vi "gbtpFit.vi"(6 "Y":dbl[](array[numeric]), 8 "error in (no error)":errorcluster, 9 "termination":cluster{"max iteration":i32, "tolerance":dbl}, 10 "X":dbl[](array[numeric]), 11 "initial parameters":dbl[](array[numeric])) -> (0 "error out":errorcluster, 1 "best nonlinear fit":dbl[](array[numeric]), 2 "covariance":T1, 3 "best fit parameters":dbl[](array[numeric]), 4 "number of function calls":i32, 5 "residue":dbl)   [LabVIEW 2021]
uses:
  <vilib>/Analysis/Matrix/Datatypes/RealMatrix.ctl
  <vilib>/gmath/NumericalOptimization/Nonlinear Curve Fit LM.vi
  <vilib>/gmath/NI_Gmath.lvlib
  <vilib>/Analysis/Matrix/NI_Matrix.lvlib
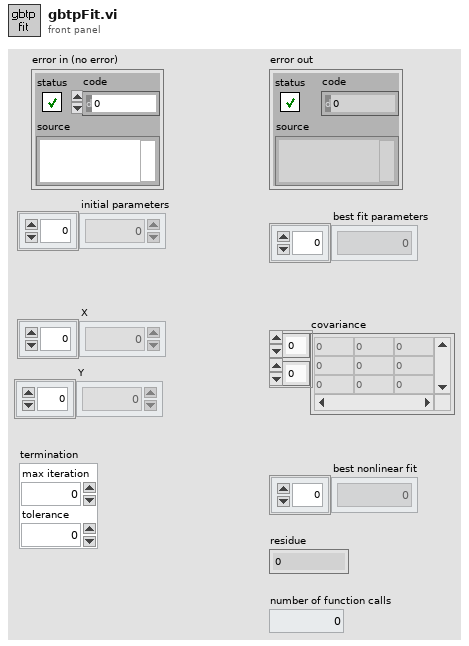
[diagram p1: front panel]
types:
  T1 = typedef "NI_Matrix.lvlib/RealMatrix.ctl" = dbl[][]
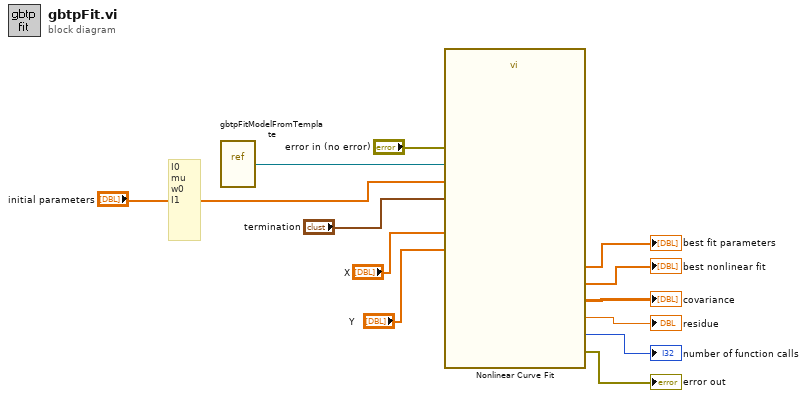
[diagram p0: block diagram]
diagram:
  # "I0\nmu\nw0\nI1"
  n1 = vi-ref "gbtpFitModelFromTemplate.vi"() -> (w6:refnum<vi>)
  n2 = call-poly <vilib>:"Nonlinear Curve Fit.vi"("Y"="Y", "f(x,a)"=w6, "X"="X", "initial parameters"="initial parameters", "error in (no error)"="error in (no error)", "termination"="termination") -> ("number of function calls"=→"number of function calls":i32, "best nonlinear fit"=→"best nonlinear fit":dbl[], "best fit parameters"=→"best fit parameters":dbl[], "covariance"=→"covariance":T1, "residue"=→"residue":dbl, "error out"=→"error out":errorcluster)  [unwired: 4 in]
